vi "Begin.vi"(8 "error in":errorcluster) -> (0 "error out":errorcluster)   [LabVIEW 2017]
doc: "Called before other user functions, this VI is expected to open initial I/O refnums, load in file data, and do all program initialization. Notice that the <B>error out</B> terminal is simply used for data flow. Wiring it to other structures or subVIs ensures that this VI runs first."
uses:
  <vilib>/Rock Robotics/WPI/DriverStation/WPI_DriverStationRobotMode2.ctl
  <vilib>/Rock Robotics/WPI/Joystick/WPI_JoystickDeviceEnum.ctl
  <vilib>/Rock Robotics/WPI/ThirdParty/Phoenix-LabVIEW/Motor Controller/Controls/CTRE_Phoenix_MotorControl_ControlMode.ctl
  <vilib>/Rock Robotics/WPI/SafetyOutput/WPI_SafetyOutputConfigMenu.ctl
  <vilib>/Rock Robotics/WPI/ThirdParty/Sensors/navX/_TypeDefs/FRIC_navX_DeviceNumbersTypeDef.ctl
  <vilib>/Rock Robotics/SystemInterfaces/AI/FPGA_AIChannel.ctl
  <vilib>/Rock Robotics/SystemInterfaces/i2clib/i2c_bus.ctl
  <vilib>/Rock Robotics/WPI/ThirdParty/Phoenix-LabVIEW/Motor Controller/Controls/CTRE_Phoenix_MotorControl_FeedbackDevice.ctl
  Robot Global Data.vi
  <vilib>/Rock Robotics/Network Tables/NT Write String Array.vi
  <vilib>/Rock Robotics/WPI/RobotDrive/WPI_RobotDriveOpen4MotorWithExistingMotors.vi
panel:
  in  "P RR":dbl=1.0
  in  "F RR":dbl=0.3074
  in  "D RR":dbl=4.0
  in  "I RR":dbl
  in  "F RF":dbl=0.3047
  in  "D RF":dbl=2.0
  in  "I RF":dbl
  in  "P RF":dbl=1.0
  in  "F LF":dbl=0.3119
  in  "D LF":dbl=4.0
  in  "I LF":dbl
  in  "P  LF":dbl=1.0
  in  "F LR":dbl=0.3074
  in  "D LR":dbl=2.0
  in  "I LR":dbl
  in  "P LR":dbl=1.0
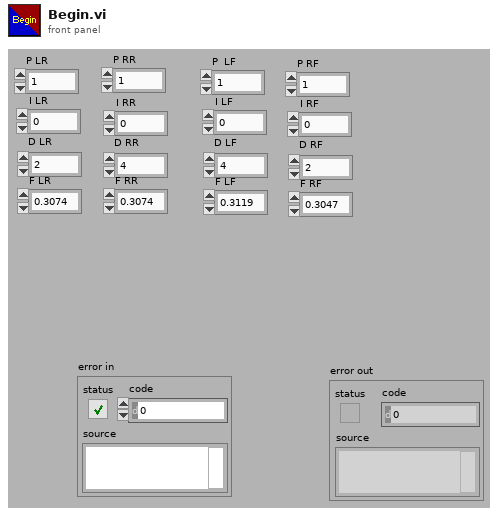
[diagram p1: front panel]
types:
  T1 = typedef "CTRE_Phoenix_MotorControl_FeedbackDevice.ctl" = i8
  T2 = typedef "i2c_bus.ctl" = enum16{"I2C On-Board", "I2C MXP", "Invalid"}
  T3 = typedef "FPGA_AIChannel.ctl" = enum8{"AI 0", "AI 1", "AI 2", "AI 3", "AI MXP 0", "AI MXP 1", "AI MXP 2", "AI MXP 3", "Invalid"}
  T4 = typedef "FRIC_navX_DeviceNumbersTypeDef.ctl" = enum16{"Dev0", "Dev1", "Dev2", "Dev3"}
  T5 = typedef "WPI_JoystickDeviceEnum.ctl" = enum16{"USB 0", "USB 1", "USB 2", "USB 3", "USB 4", "USB 5"}
  T6 = typedef "WPI_SafetyOutputConfigMenu.ctl" = enum16{"Enable", "Disable"}
  T7 = typedef "CTRE_Phoenix_MotorControl_ControlMode.ctl" = u16
  T8 = typedef "WPI_DriverStationRobotMode2.ctl" = enum16{"Autonomous Disabled", "Autonomous Enabled", "Teleop Disabled", "Teleop Enabled", "Disconnected", "Finish", "Test Disabled", "Test Enabled", "Emergency Stopped"}
  T9 = typedef "WPI_MotorControlDeviceRef.ctl" = cluster{"DeviceStatus":errorcluster, "Type":T10, "PWM":cluster{"PWM Channel":T11, "DeadBand":T12}, "CAN":cluster{"Device Number":u8, "SetOutput VI Ref":variant, "GetOutput VI Ref":variant, "Enable VI Ref":variant, "Disable VI Ref":variant, "Data":variant}, "Invert":bool, "DIO PWM":cluster{"PWM \"Enable\" Channel":T11, "DIOChannel":T13, "PWM Rate":dbl}}
  T10 = typedef "WPI_MotorControlType.ctl" = enum16{"PWM", "CAN", "DIO PWM"}
  T11 = typedef "FPGA_DIOPWMChannel.ctl" = enum8{"PWM 0", "PWM 1", "PWM 2", "PWM 3", "PWM 4", "PWM 5", "PWM 6", "PWM 7", "PWM 8", "PWM 9", "PWM MXP 0", "PWM MXP 1", "PWM MXP 2", "PWM MXP 3", "PWM MXP 4", "PWM MXP 5", "PWM MXP 6", "PWM MXP 7", "PWM MXP 8", "PWM MXP 9", "Invalid"}
  T12 = typedef "WPI_PWMDeadband.ctl" = cluster{"Name":string, "maxPositivePwm":i32, "minPositivePwm":i32, "centerPwm":i32, "maxNegativePwm":i32, "minNegativePwm":i32, "angularRange":u16}
  T13 = typedef "FPGA_DIOChannel.ctl" = enum8{"DIO 0", "DIO 1", "DIO 2", "DIO 3", "DIO 4", "DIO 5", "DIO 6", "DIO 7", "DIO 8", "DIO 9", "DIO MXP 0", "DIO MXP 1", "DIO MXP 2", "DIO MXP 3", "DIO MXP 4", "DIO MXP 5", "DIO MXP 6", "DIO MXP 7", "DIO MXP 8", "DIO MXP 9", "DIO MXP 10", "DIO MXP 11", "DIO MXP 12", "DIO MXP 13", "DIO MXP 14", "DIO MXP 15", "SPI Port CS1", "SPI Port CS2", "SPI Port CS3", "SPI Port MISO", "SPI Port MOSI", "Invalid"}
  T14 = typedef "WPI_AnalogChannelDevRef.ctl" = cluster{"DevStatus":errorcluster, "Analog Channel":T3}
  T15 = typedef "WPI_I2CDevRef.ctl" = cluster{"DevStatus":errorcluster, "Device Address":u8, "Handle":i32, "I2C Bus":T2}
  T16 = typedef "WPI_JoystickDevRef.ctl" = cluster{"Device":T5}
  T17 = typedef "WPI_RobotDriveDevRef.ctl" = cluster{"DevStatus":errorcluster, "Motors[]":T9[], "Square Inputs":bool, "Max Output":dbl}
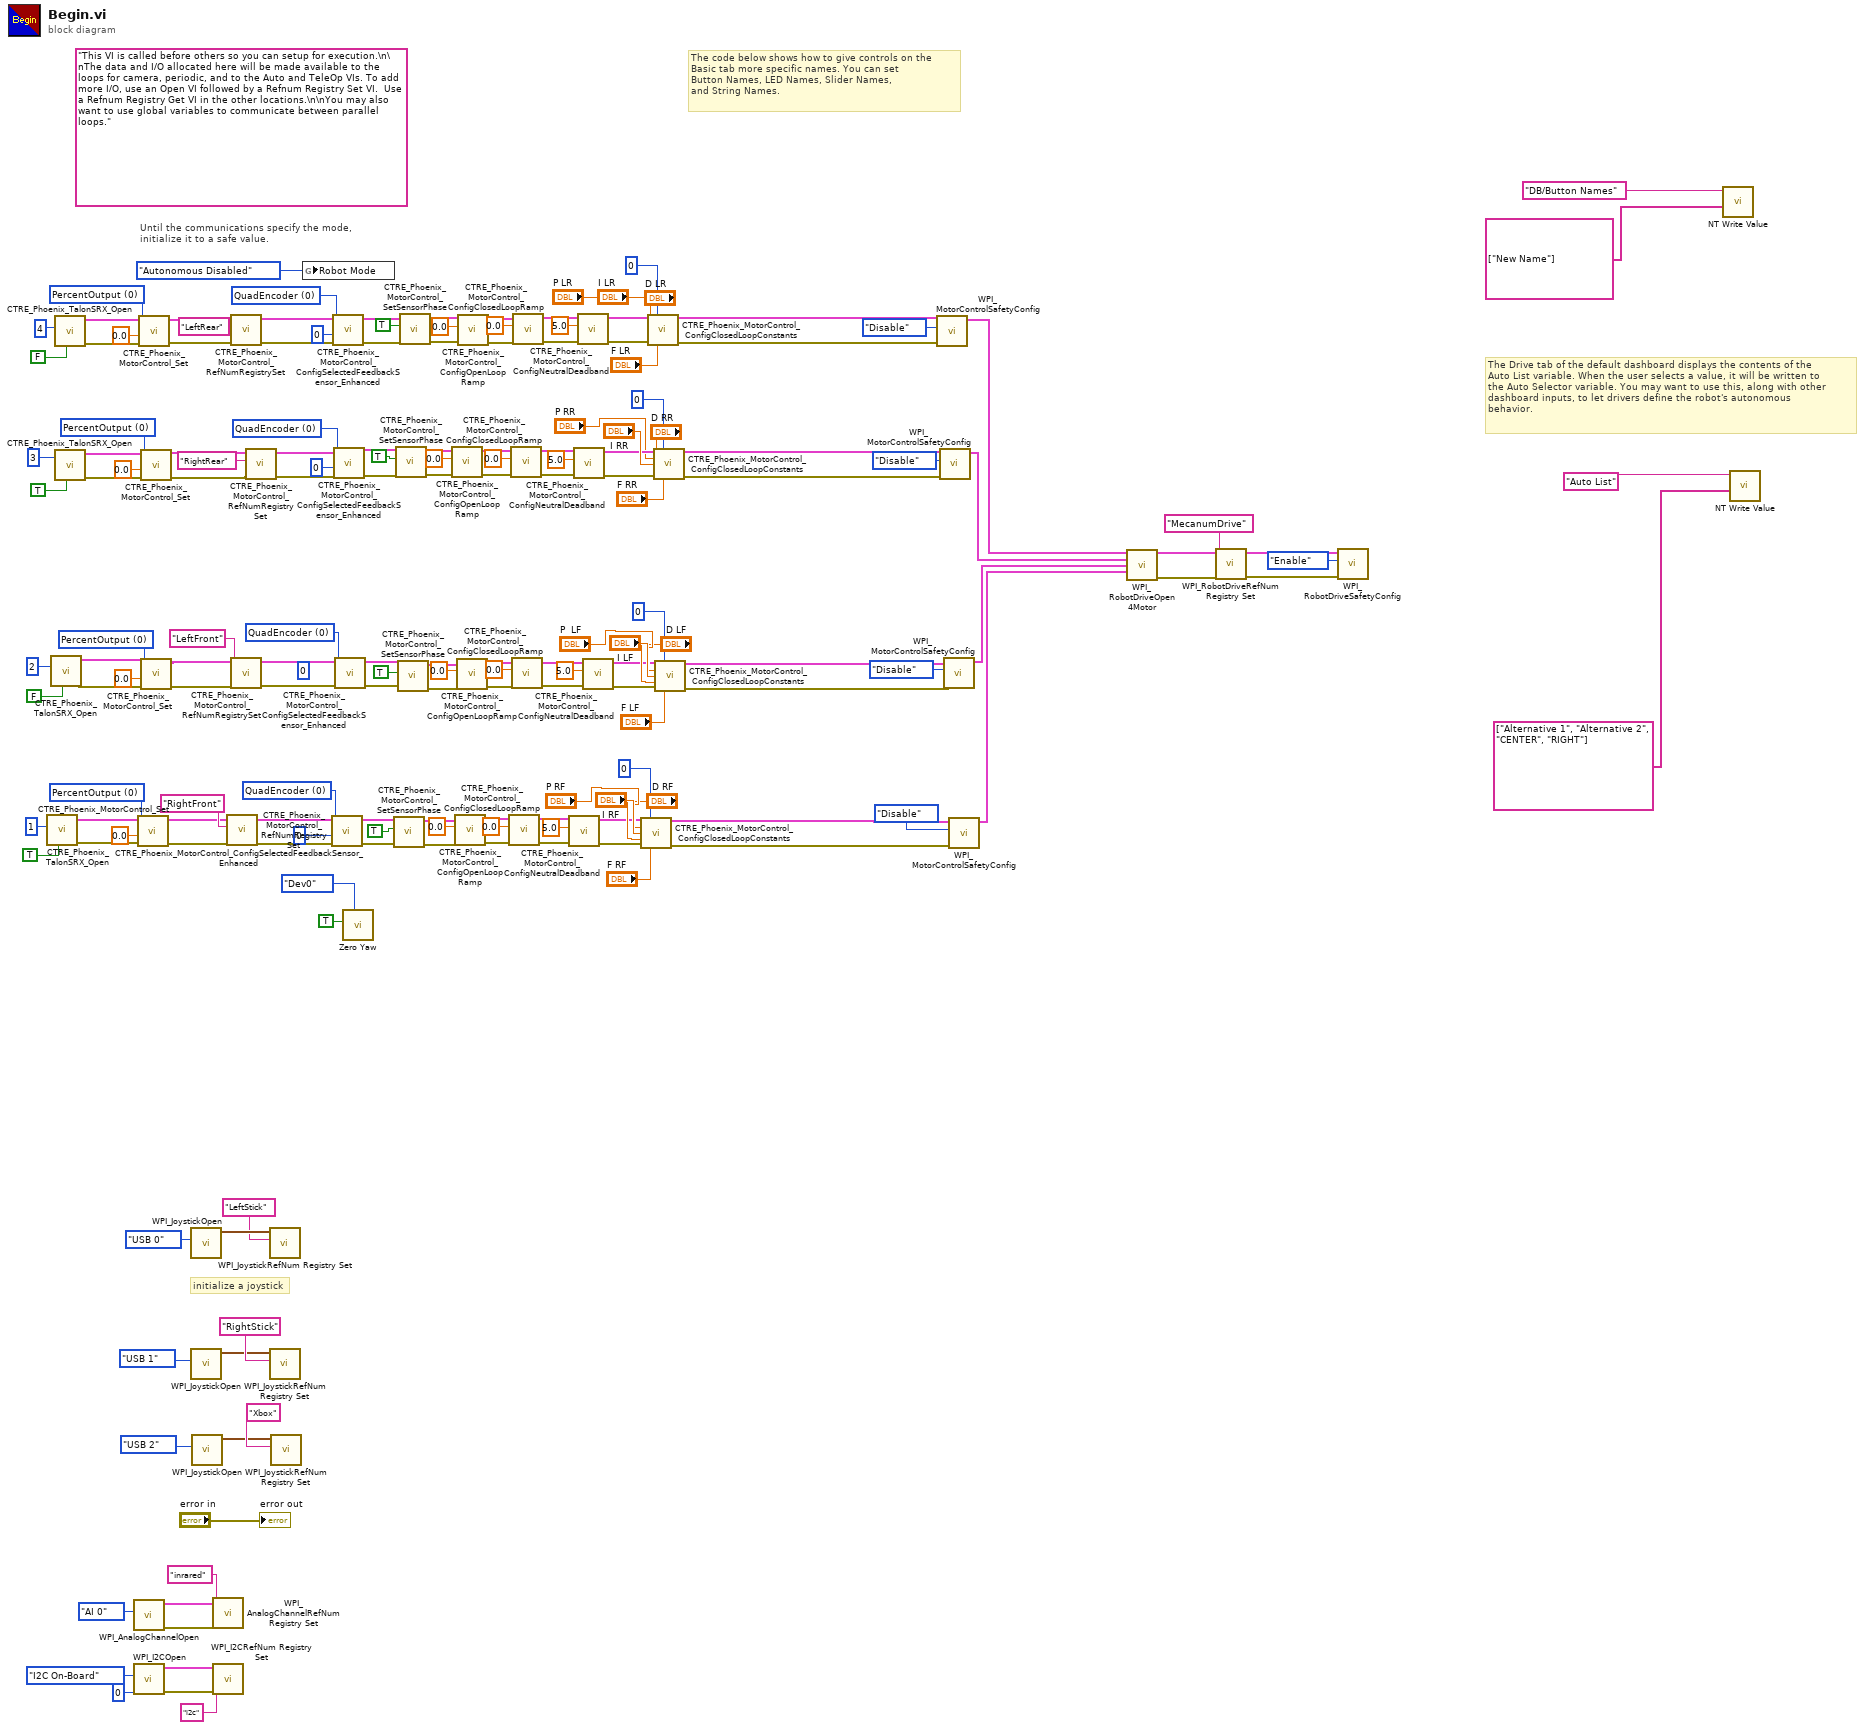
[diagram p0: block diagram]
diagram:
  w92 = T1 0 items=["None"=-1, "QuadEncoder"=0, "Analog"=2, "Tachometer"=4, "Pulse Width Encoded Position"=8, "Sensor Sum (S0 + S1)"=9, "Sensor Difference (D0 - D1)"=10, "Remote Source 0"=11, "Remote Source 1"=12, "Software Emulated"=15] ("Feedback Device")
  (unwired) 0 ("pidLoopIdx")
  w95 = T1 0 items=["None"=-1, "QuadEncoder"=0, "Analog"=2, "Tachometer"=4, "Pulse Width Encoded Position"=8, "Sensor Sum (S0 + S1)"=9, "Sensor Difference (D0 - D1)"=10, "Remote Source 0"=11, "Remote Source 1"=12, "Software Emulated"=15] ("Feedback Device")
  w99 = T1 0 items=["None"=-1, "QuadEncoder"=0, "Analog"=2, "Tachometer"=4, "Pulse Width Encoded Position"=8, "Sensor Sum (S0 + S1)"=9, "Sensor Difference (D0 - D1)"=10, "Remote Source 0"=11, "Remote Source 1"=12, "Software Emulated"=15] ("Feedback Device")
  w101 = T1 0 items=["None"=-1, "QuadEncoder"=0, "Analog"=2, "Tachometer"=4, "Pulse Width Encoded Position"=8, "Sensor Sum (S0 + S1)"=9, "Sensor Difference (D0 - D1)"=10, "Remote Source 0"=11, "Remote Source 1"=12, "Software Emulated"=15] ("Feedback Device")
  w157 = T7 0 items=["PercentOutput"=0, "Position"=1, "Velocity"=2, "Current"=3, "Follower"=5, "MotionProfile"=6, "MotionMagic"=7, "MotionMagicArc"=8, "MotionProfileArc"=10, "Disabled"=15] ("Control Mode")
  w158 = T7 0 items=["PercentOutput"=0, "Position"=1, "Velocity"=2, "Current"=3, "Follower"=5, "MotionProfile"=6, "MotionMagic"=7, "MotionMagicArc"=8, "MotionProfileArc"=10, "Disabled"=15] ("Control Mode")
  w159 = T7 0 items=["PercentOutput"=0, "Position"=1, "Velocity"=2, "Current"=3, "Follower"=5, "MotionProfile"=6, "MotionMagic"=7, "MotionMagicArc"=8, "MotionProfileArc"=10, "Disabled"=15] ("Control Mode")
  w160 = T7 0 items=["PercentOutput"=0, "Position"=1, "Velocity"=2, "Current"=3, "Follower"=5, "MotionProfile"=6, "MotionMagic"=7, "MotionMagicArc"=8, "MotionProfileArc"=10, "Disabled"=15] ("Control Mode")
  (unwired) "This VI is called before others so you can setup for execution.\n\nThe data and I/O allocated here will be made available to the loops for camera, periodic, and to the Auto and TeleOp VIs. To add more I/O, use an Open VI followed by a Refnum Registry Set VI.  Use a Refnum Registry Get VI in the other locations.\n\nYou may also want to use global variables to communicate between parallel loops."
  # "initialize a joystick"
  # "The Drive tab of the default dashboard displays the contents of the\nAuto List variable. When the user selects a value, it will be written to\nthe Auto Selector variable. You may want to use this, along with other\ndashboard inputs, to let drivers define the robot's autonomous\nbehavior."
  # "The code below shows how to give controls on the\nBasic tab more specific names. You can set\nButton Names, LED Names, Slider Names,\nand String Names."
  # "Until the communications specify the mode,\ninitialize it to a safe value."
  n1 = call <vilib>:"CTRE_Phoenix_TalonSRX_Open.vi"("Invert"=TRUE, "Device Number"=u8 1) -> ("error out"=w151:errorcluster, "CAN Talon SRX Ref"=w152:T9)  [unwired: 8 in]
  n2 = call <vilib>:"CTRE_Phoenix_TalonSRX_Open.vi"("Invert"=FALSE, "Device Number"=u8 2) -> ("error out"=w153:errorcluster, "CAN Talon SRX Ref"=w154:T9)  [unwired: 8 in]
  n3 = call <vilib>:"CTRE_Phoenix_TalonSRX_Open.vi"("Invert"=FALSE, "Device Number"=u8 4) -> ("error out"=w161:errorcluster, "CAN Talon SRX Ref"=w162:T9)  [unwired: 8 in]
  n4 = call <vilib>:"CTRE_Phoenix_TalonSRX_Open.vi"("Invert"=TRUE, "Device Number"=u8 3) -> ("error out"=w155:errorcluster, "CAN Talon SRX Ref"=w156:T9)  [unwired: 8 in]
  n5 = call <vilib>:"WPI_AnalogChannelOpen.vi"("Analog Channel"=FPGA_AIChannel."AI 0") -> ("error out"=w110:errorcluster, "AIDeviceRef"=w111:T14)  [unwired: 9 in]
  n6 = call <vilib>:"WPI_I2COpen.vi"("Device Address"=u8 0, "I2C Bus"=i2c_bus."I2C On-Board") -> ("error out"=w105:errorcluster, "I2CDevRef"=w106:T15)  [unwired: 8 in]
  n7 = call <vilib>:"CTRE_Phoenix_MotorControl_Set.vi"("error in (no error)"=w151, "Output"=0.0, "Control Mode"=w157, "PhoenixMotorControlDevRef"=w152) -> ("error out"=w139:errorcluster, "PhoenixMotorControlDevRef"=w140:T9)  [unwired: 6 in]
  n8 = call <vilib>:"CTRE_Phoenix_MotorControl_Set.vi"("error in (no error)"=w161, "Output"=0.0, "Control Mode"=w160, "PhoenixMotorControlDevRef"=w162) -> ("error out"=w149:errorcluster, "PhoenixMotorControlDevRef"=w150:T9)  [unwired: 6 in]
  n9 = call <vilib>:"CTRE_Phoenix_MotorControl_Set.vi"("error in (no error)"=w155, "Output"=0.0, "Control Mode"=w159, "PhoenixMotorControlDevRef"=w156) -> ("error out"=w141:errorcluster, "PhoenixMotorControlDevRef"=w142:T9)  [unwired: 6 in]
  n10 = call <vilib>:"CTRE_Phoenix_MotorControl_Set.vi"("error in (no error)"=w153, "Output"=0.0, "Control Mode"=w158, "PhoenixMotorControlDevRef"=w154) -> ("error out"=w143:errorcluster, "PhoenixMotorControlDevRef"=w144:T9)  [unwired: 6 in]
  n11 = call <vilib>:"WPI_JoystickOpen.vi"("JoystickDevice"=WPI_JoystickDeviceEnum."USB 0") -> ("JoystickDevRef"=w128:T16)  [unwired: 10 in]
  n12 = call <vilib>:"WPI_JoystickOpen.vi"("JoystickDevice"=WPI_JoystickDeviceEnum."USB 1") -> ("JoystickDevRef"=w173:T16)  [unwired: 10 in]
  n13 = call <vilib>:"WPI_JoystickOpen.vi"("JoystickDevice"=WPI_JoystickDeviceEnum."USB 2") -> ("JoystickDevRef"=w118:T16)  [unwired: 10 in]
  n14 = call <vilib>:"WPI_AnalogChannelRefNum Registry Set.vi"("error in (no error)"=w110, "refnum name"="inrared", "AIDeviceRef"=w111) -> ()  [unwired: 7 in, 2 out]
  n15 = call <vilib>:"WPI_I2CRefNum Registry Set.vi"("error in (no error)"=w105, "refnum name"="i2c", "I2CDevRef"=w106) -> ()  [unwired: 7 in, 2 out]
  n16 = call <vilib>:"CTRE_Phoenix_MotorControl_RefNumRegistrySet.vi"("error in (no error)"=w139, "refnum name"="RightFront", "PhoenixMotorControlDevRef"=w140) -> ("error out"=w90:errorcluster, "PhoenixMotorControlDevRef"=w91:T9)  [unwired: 7 in]
  n17 = call <vilib>:"CTRE_Phoenix_MotorControl_RefNumRegistrySet.vi"("error in (no error)"=w149, "refnum name"="LeftRear", "PhoenixMotorControlDevRef"=w150) -> ("error out"=w102:errorcluster, "PhoenixMotorControlDevRef"=w103:T9)  [unwired: 7 in]
  n18 = call <vilib>:"CTRE_Phoenix_MotorControl_RefNumRegistrySet.vi"("error in (no error)"=w143, "refnum name"="LeftFront", "PhoenixMotorControlDevRef"=w144) -> ("error out"=w94:errorcluster, "PhoenixMotorControlDevRef"=w93:T9)  [unwired: 7 in]
  n19 = call <vilib>:"CTRE_Phoenix_MotorControl_RefNumRegistrySet.vi"("error in (no error)"=w141, "refnum name"="RightRear", "PhoenixMotorControlDevRef"=w142) -> ("error out"=w96:errorcluster, "PhoenixMotorControlDevRef"=w97:T9)  [unwired: 7 in]
  n20 = call <vilib>:"WPI_JoystickRefNum Registry Set.vi"("refnum name"="LeftStick", "JoystickDevRef"=w128) -> ()  [unwired: 8 in, 2 out]
  n21 = call <vilib>:"WPI_JoystickRefNum Registry Set.vi"("refnum name"="RightStick", "JoystickDevRef"=w173) -> ()  [unwired: 8 in, 2 out]
  n22 = call <vilib>:"WPI_JoystickRefNum Registry Set.vi"("refnum name"="Xbox", "JoystickDevRef"=w118) -> ()  [unwired: 8 in, 2 out]
  n23 = global write "Robot Global Data.vi" "Robot Mode"(WPI_DriverStationRobotMode2."Autonomous Disabled" ("Robot Mode")) -> ()
  n24 = call <vilib>:"CTRE_Phoenix_MotorControl_ConfigSelectedFeedbackSensor_Enhanced.vi"("error in (no error)"=w90, "pidLoopIdx"=0, "Feedback Device"=w92, "PhoenixMotorControlDevRef"=w91) -> ("error out"=w81:errorcluster, "PhoenixMotorControlDevRef"=w82:T9)  [unwired: 6 in]
  n25 = call <vilib>:"CTRE_Phoenix_MotorControl_ConfigSelectedFeedbackSensor_Enhanced.vi"("error in (no error)"=w102, "pidLoopIdx"=0, "Feedback Device"=w101, "PhoenixMotorControlDevRef"=w103) -> ("error out"=w87:errorcluster, "PhoenixMotorControlDevRef"=w88:T9)  [unwired: 6 in]
  n26 = call <vilib>:"CTRE_Phoenix_MotorControl_ConfigSelectedFeedbackSensor_Enhanced.vi"("error in (no error)"=w96, "pidLoopIdx"=0, "Feedback Device"=w99, "PhoenixMotorControlDevRef"=w97) -> ("error out"=w78:errorcluster, "PhoenixMotorControlDevRef"=w77:T9)  [unwired: 6 in]
  n27 = call <vilib>:"CTRE_Phoenix_MotorControl_ConfigSelectedFeedbackSensor_Enhanced.vi"("error in (no error)"=w94, "Feedback Device"=w95, "PhoenixMotorControlDevRef"=w93) -> ("error out"=w80:errorcluster, "PhoenixMotorControlDevRef"=w79:T9)  [unwired: 7 in]
  n28 = call <vilib>:"Zero Yaw.vi"("Device Number"=FRIC_navX_DeviceNumbersTypeDef."Dev0", "Zero"=TRUE) -> ()  [unwired: 10 in]
  n29 = call <vilib>:"CTRE_Phoenix_MotorControl_SetSensorPhase.vi"("error in (no error)"=w81, "PhaseSensor"=TRUE, "PhoenixMotorControlDevRef"=w82) -> ("error out"=w69:errorcluster, "PhoenixMotorControlDevRef"=w70:T9)  [unwired: 7 in]
  n30 = call <vilib>:"CTRE_Phoenix_MotorControl_SetSensorPhase.vi"("error in (no error)"=w78, "PhaseSensor"=TRUE, "PhoenixMotorControlDevRef"=w77) -> ("error out"=w73:errorcluster, "PhoenixMotorControlDevRef"=w74:T9)  [unwired: 7 in]
  n31 = call <vilib>:"CTRE_Phoenix_MotorControl_SetSensorPhase.vi"("error in (no error)"=w80, "PhaseSensor"=TRUE, "PhoenixMotorControlDevRef"=w79) -> ("error out"=w71:errorcluster, "PhoenixMotorControlDevRef"=w72:T9)  [unwired: 7 in]
  n32 = call <vilib>:"CTRE_Phoenix_MotorControl_SetSensorPhase.vi"("error in (no error)"=w87, "PhaseSensor"=TRUE, "PhoenixMotorControlDevRef"=w88) -> ("error out"=w75:errorcluster, "PhoenixMotorControlDevRef"=w76:T9)  [unwired: 7 in]
  n33 = call <vilib>:"CTRE_Phoenix_MotorControl_ConfigOpenLoopRamp.vi"("error in (no error)"=w73, "secondsFromNeutralToFull"=0.0, "PhoenixMotorControlDevRef"=w74) -> ("error out"=w63:errorcluster, "PhoenixMotorControlDevRef"=w64:T9)  [unwired: 7 in]
  n34 = call <vilib>:"CTRE_Phoenix_MotorControl_ConfigOpenLoopRamp.vi"("error in (no error)"=w69, "secondsFromNeutralToFull"=0.0, "PhoenixMotorControlDevRef"=w70) -> ("error out"=w65:errorcluster, "PhoenixMotorControlDevRef"=w66:T9)  [unwired: 7 in]
  n35 = call <vilib>:"CTRE_Phoenix_MotorControl_ConfigOpenLoopRamp.vi"("error in (no error)"=w71, "secondsFromNeutralToFull"=0.0, "PhoenixMotorControlDevRef"=w72) -> ("error out"=w67:errorcluster, "PhoenixMotorControlDevRef"=w68:T9)  [unwired: 7 in]
  n36 = call <vilib>:"CTRE_Phoenix_MotorControl_ConfigOpenLoopRamp.vi"("error in (no error)"=w75, "secondsFromNeutralToFull"=0.0, "PhoenixMotorControlDevRef"=w76) -> ("error out"=w62:errorcluster, "PhoenixMotorControlDevRef"=w61:T9)  [unwired: 7 in]
  n37 = call <vilib>:"CTRE_Phoenix_MotorControl_ConfigClosedLoopRamp.vi"("error in (no error)"=w65, "secondsFromNeutralToFull"=0.0, "PhoenixMotorControlDevRef"=w66) -> ("error out"=w23:errorcluster, "PhoenixMotorControlDevRef"=w24:T9)  [unwired: 7 in]
  n38 = call <vilib>:"CTRE_Phoenix_MotorControl_ConfigClosedLoopRamp.vi"("error in (no error)"=w63, "secondsFromNeutralToFull"=0.0, "PhoenixMotorControlDevRef"=w64) -> ("error out"=w48:errorcluster, "PhoenixMotorControlDevRef"=w49:T9)  [unwired: 7 in]
  n39 = call <vilib>:"CTRE_Phoenix_MotorControl_ConfigClosedLoopRamp.vi"("error in (no error)"=w67, "secondsFromNeutralToFull"=0.0, "PhoenixMotorControlDevRef"=w68) -> ("error out"=w32:errorcluster, "PhoenixMotorControlDevRef"=w33:T9)  [unwired: 7 in]
  n40 = call <vilib>:"CTRE_Phoenix_MotorControl_ConfigClosedLoopRamp.vi"("error in (no error)"=w62, "secondsFromNeutralToFull"=0.0, "PhoenixMotorControlDevRef"=w61) -> ("error out"=w51:errorcluster, "PhoenixMotorControlDevRef"=w52:T9)  [unwired: 7 in]
  n41 = call <vilib>:"CTRE_Phoenix_MotorControl_ConfigNeutralDeadband.vi"("error in (no error)"=w23, "Percent Deadband"=5.0, "PhoenixMotorControlDevRef"=w24) -> ("error out"=w25:errorcluster, "PhoenixMotorControlDevRef"=w26:T9)  [unwired: 7 in]
  n42 = call <vilib>:"CTRE_Phoenix_MotorControl_ConfigNeutralDeadband.vi"("error in (no error)"=w48, "Percent Deadband"=5.0, "PhoenixMotorControlDevRef"=w49) -> ("error out"=w4:errorcluster, "PhoenixMotorControlDevRef"=w5:T9)  [unwired: 7 in]
  n43 = call <vilib>:"CTRE_Phoenix_MotorControl_ConfigNeutralDeadband.vi"("error in (no error)"=w51, "Percent Deadband"=5.0, "PhoenixMotorControlDevRef"=w52) -> ("error out"=w45:errorcluster, "PhoenixMotorControlDevRef"=w46:T9)  [unwired: 7 in]
  n44 = call <vilib>:"CTRE_Phoenix_MotorControl_ConfigNeutralDeadband.vi"("error in (no error)"=w32, "Percent Deadband"=5.0, "PhoenixMotorControlDevRef"=w33) -> ("error out"=w34:errorcluster, "PhoenixMotorControlDevRef"=w35:T9)  [unwired: 7 in]
  n45 = call <vilib>:"CTRE_Phoenix_MotorControl_ConfigClosedLoopConstants.vi"("PhoenixMotorControlDevRef"=w26, "slotIdx"=0, "P"="P RF", "I"="I RF", "D"="D RF", "error in (no error)"=w25, "F"="F RF") -> ("PhoenixMotorControlDevRef"=w15:T9, "error out"=w14:errorcluster)  [unwired: 7 in]
  n46 = call <vilib>:"CTRE_Phoenix_MotorControl_ConfigClosedLoopConstants.vi"("PhoenixMotorControlDevRef"=w46, "slotIdx"=0, "P"="P LR", "I"="I LR", "D"="D LR", "error in (no error)"=w45, "F"="F LR") -> ("PhoenixMotorControlDevRef"=w19:T9, "error out"=w18:errorcluster)  [unwired: 7 in]
  n47 = call <vilib>:"CTRE_Phoenix_MotorControl_ConfigClosedLoopConstants.vi"("PhoenixMotorControlDevRef"=w5, "slotIdx"=0, "P"="P RR", "I"="I RR", "D"="D RR", "error in (no error)"=w4, "F"="F RR") -> ("PhoenixMotorControlDevRef"=w2:T9, "error out"=w1:errorcluster)  [unwired: 7 in]
  n48 = call <vilib>:"CTRE_Phoenix_MotorControl_ConfigClosedLoopConstants.vi"("PhoenixMotorControlDevRef"=w35, "slotIdx"=0, "P"="P  LF", "I"="I LF", "D"="D LF", "error in (no error)"=w34, "F"="F LF") -> ("PhoenixMotorControlDevRef"=w17:T9, "error out"=w16:errorcluster)  [unwired: 7 in]
  n49 = call <vilib>:"WPI_MotorControlSafetyConfig.vi"("error in (no error)"=w18, "mode"=WPI_SafetyOutputConfigMenu."Disable", "MotorControlDevRef"=w19) -> ("MotorControlDevRef"=w13:T9)  [unwired: 7 in, 1 out]
  n50 = call <vilib>:"WPI_MotorControlSafetyConfig.vi"("error in (no error)"=w1, "mode"=WPI_SafetyOutputConfigMenu."Disable", "MotorControlDevRef"=w2) -> ("MotorControlDevRef"=w12:T9)  [unwired: 7 in, 1 out]
  n51 = call <vilib>:"WPI_MotorControlSafetyConfig.vi"("error in (no error)"=w16, "mode"=WPI_SafetyOutputConfigMenu."Disable", "MotorControlDevRef"=w17) -> ("MotorControlDevRef"=w11:T9)  [unwired: 7 in, 1 out]
  n52 = call <vilib>:"WPI_MotorControlSafetyConfig.vi"("error in (no error)"=w14, "mode"=WPI_SafetyOutputConfigMenu."Disable", "MotorControlDevRef"=w15) -> ("MotorControlDevRef"=w10:T9)  [unwired: 7 in, 1 out]
  n53 = call-poly <vilib>:"WPI_RobotDriveOpen4Motor.vi"("Rear Left Motor Dev Ref"=w13, "Rear Right Motor Dev Ref"=w12, "Front Left Motor Dev Ref"=w11, "Front Right Motor Dev Ref"=w10) -> ("RobotDriveDevRef"=w138:T17, "error out"=w137:errorcluster)  [unwired: 10 in]
  n54 = call <vilib>:"WPI_RobotDriveRefNum Registry Set.vi"("error in (no error)"=w137, "refnum name"="MecanumDrive", "RobotDriveDevRef"=w138) -> ("error out"=w134:errorcluster, "RobotDriveDevRef"=w135:T17)  [unwired: 7 in]
  n55 = call <vilib>:"WPI_RobotDriveSafetyConfig.vi"("error in (no error)"=w134, "mode"=WPI_SafetyOutputConfigMenu."Enable", "RobotDriveDevRef"=w135) -> ()  [unwired: 7 in, 2 out]
  n56 = call-poly <vilib>:"NT Write Value.vi"("String Array"=string[] ["New Name"], "Name"="DB/Button Names") -> ()  [unwired: 9 in, 1 out]
  n57 = call-poly <vilib>:"NT Write Value.vi"("String Array"=string[] ["Alternative 1", "Alternative 2", "CENTER", "RIGHT"], "Name"="Auto List") -> ()  [unwired: 9 in, 1 out]
  "error out" <- "error in"
